vi "SandwitchingValues.vi"(8 "DesiredAngle":dbl, 10 "Angle Array":dbl[](array[numeric])) -> (3 "Angle Indexes":dbl[](array[numeric]))   [LabVIEW 2012, in "LinearInterpolation.lvclass"]
doc: "Determines indecies of angles in the input array sandwitching the desired Array"
uses:
  LinearInterpolation.lvclass
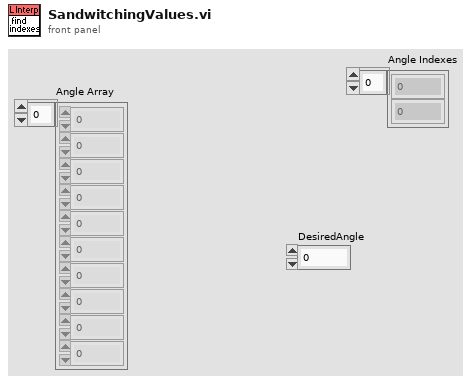
[diagram p1: front panel]
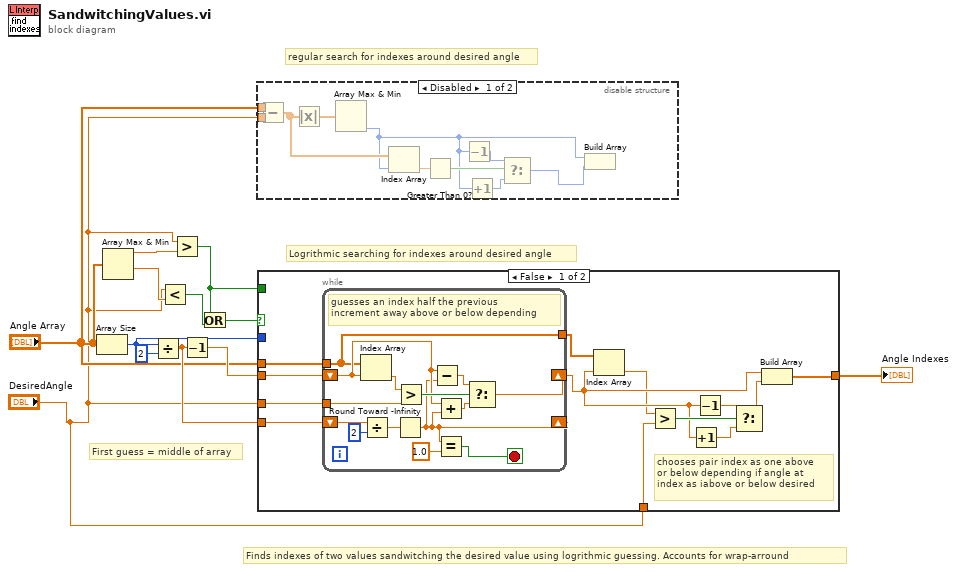
[diagram p0: block diagram]
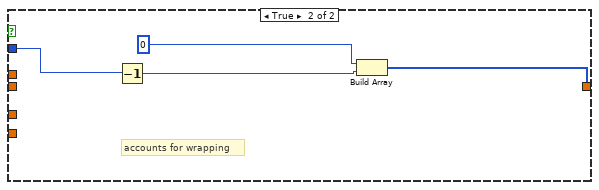
[diagram p2: hidden frame]
diagram:
  # "regular search for indexes around desired angle"
  # "Logrithmic searching for indexes around desired angle"
  # "First guess = middle of array"
  # "Finds indexes of two values sandwitching the desired value using logrithmic guessing. Accounts for wrap-arround"
  n1 = Array Size(array="Angle Array") -> (size(s)=w6:i32)
  n2 = Array Max & Min(array="Angle Array") -> (max value=w2:dbl, min value=w4:dbl)  [unwired: 2 out]
  n3 = Divide(x=w6, y=2) -> (x/y=w10:dbl)
  n4 = Less?(x="DesiredAngle", y=w4) -> (x < y?=w7:bool)
  n5 = Greater?(x="DesiredAngle", y=w2) -> (0:w3:bool)
  n6 = Decrement(x=w10) -> (x-1=w11:dbl)
  n7 = Or(x=w3, y=w7) -> (x .or. y?=w9:bool)
  n8 = disable-structure shown="Disabled" {
    disable-tunnel: "Angle Array" -> [w14 _]
    disable-tunnel: "DesiredAngle" -> [w13 _]
    frame Disabled {
      n9 = Subtract(x=w14, y=w13) -> (x-y=w22:dbl[])
      n10 = Absolute Value(x=w22) -> (abs(x)=w23:dbl[])
      n11 = Array Max & Min(array=w23) -> (min index (indices)=w17:i32)  [unwired: 3 out]
      n12 = Index Array(array=w22, index=w17) -> (element=w21:dbl)
      n13 = Greater Than 0?(x=w21) -> (x > 0?=w20:bool)
      n14 = Decrement(x=w17) -> (x-1=w18:i32)
      n15 = Increment(x=w17) -> (x+1=w19:i32)
      n16 = Select(t=w18, s=w20, f=w19) -> (s? t:f=w16:i32)
      n17 = Build Array(w17, w16) -> (w15:i32[])
    }
    frame Enabled {
    }
  }
  n18 = case shown="False" w9 {
    tunnel: "Angle Array" -> [w36 _]
    tunnel: w11 -> [w35 _]
    tunnel: w10 -> [w34 _]
    tunnel: "DesiredAngle" -> [w33 _]
    tunnel: [w28 w51] -> w5
    tunnel: w3 -> [_ _]
    tunnel: w6 -> [_ w54]
    tunnel: "DesiredAngle" -> [w24 _]
    frame False {
      # "chooses pair index as one above  \nor below depending if angle at \nindex as iabove or below desired"
      n19 = while {
        tunnel: w36 -> [w37]
        tunnel: w33 -> [w49]
        shift-right: [w44] -> w26
        shift-left: w35 -> [w45]
        shift-right: [w38] -> _
        shift-left: w34 -> [w41]
        tunnel: [w37] -> w27
        stop <- w39 stop-if-true
        # "guesses an index half the previous \nincrement away above or below depending"
        n20 = Index Array(array=w37, index=w45) -> (element=w50:dbl)
        n21 = Divide(x=w41, y=2) -> (x/y=w43:dbl)
        n22 = Round Toward -Infinity(1:w43) -> (0:w38:dbl)
        n23 = Greater?(x=w50, y=w49) -> (0:w48:bool)
        n24 = Subtract(x=w45, y=w38) -> (x-y=w47:dbl)
        n25 = Add(x=w45, y=w38) -> (x+y=w46:dbl)
        n26 = Equal?(x=w38, y=1.0) -> (x = y?=w39:bool)
        n27 = Select(t=w47, s=w48, f=w46) -> (s? t:f=w44:dbl)
      }
      n28 = Index Array(array=w27, index=w26) -> (element=w25:dbl)
      n29 = Greater?(x=w25, y=w24) -> (0:w32:bool)
      n30 = Increment(x=w26) -> (x+1=w30:dbl)
      n31 = Decrement(x=w26) -> (x-1=w31:dbl)
      n32 = Select(t=w31, s=w32, f=w30) -> (s? t:f=w29:dbl)
      n33 = Build Array(w26, w29) -> (w28:dbl[])
    }
    frame True {
      # "accounts for wrapping"
      n34 = Decrement(x=w54) -> (x-1=w52:i32)
      n35 = Build Array(0 ("t"), w52) -> (w51:i32[])
    }
  }
  "Angle Indexes" <- w5
